vi "DT_Find Next Triangulation_Base Point.vi"(7 "left/right pt (right:F)":bool, 8 "search point":i32, 9 "external point":i32, 10 "Triangles In":i32[][](array[numeric]), 11 "Points In":cluster{"x":dbl, "y":dbl, "index":i32}[](array[cluster])) -> (0 "base point":i32, 1 "triangle":i32, 2 "Triangles Out":i32[][](array[numeric]), 3 "Points Out":cluster{"x":dbl, "y":dbl, "index":i32}[](array[cluster]), 4 "error":i32)   [LabVIEW 2017, in "NI_AAL_Geometry.lvlib"]
uses:
  <vilib>/Analysis/NI_AAL_Geometry.lvlib
  <vilib>/Analysis/geometry.llb/DT_Triangle Manager_Get Adj_by Point.vi
  <vilib>/Analysis/geometry.llb/DT_Triangle Manager_Get Oppo Point_in Ghost.vi
  <vilib>/Analysis/geometry.llb/DT_Triangle Manager_Get Ghost Point.vi
  <vilib>/Analysis/geometry.llb/DT_Triangle Manager_Get Oppo Point.vi
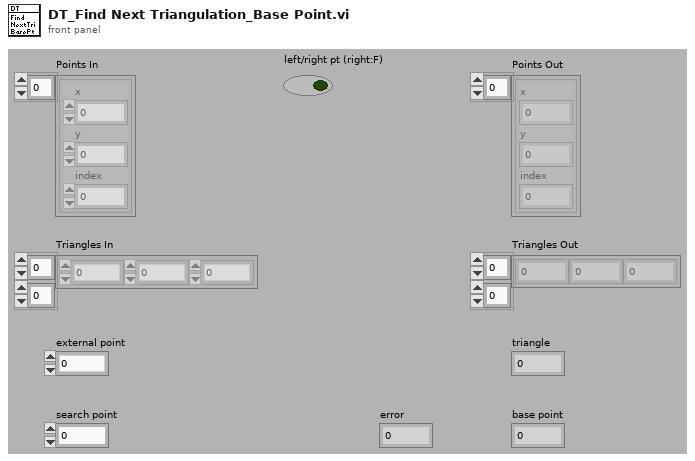
[diagram p1: front panel]
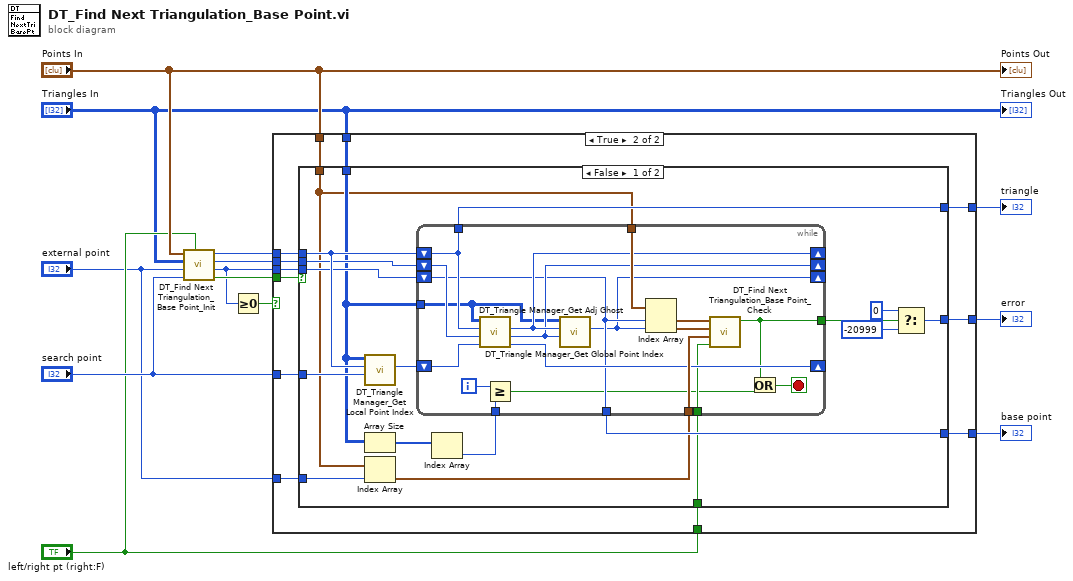
[diagram p0: block diagram]
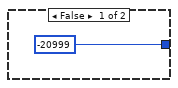
[diagram p2: hidden frame]
diagram:
  n1 = call <vilib>:"DT_Find Next Triangulation_Base Point_Init.vi"("left/right pt (right:F)"="left/right pt (right:F)", "search point"="search point", "external point"="external point", "Triangles In"="Triangles In", "Points In"="Points In") -> ("done?"=w11:bool, "global idx"=w2:i32, "local idx"=w9:i32, "triangle"=w10:i32)  [unwired: 3 in]
  n2 = Greater Or Equal To 0?(x=w2) -> (x >= 0?=w1:bool)
  n3 = case shown="True" w1 {
    tunnel: [_ w26] -> w13
    tunnel: [_ w25] -> w12
    tunnel: w11 -> [_ w24]
    tunnel: w10 -> [_ w23]
    tunnel: w9 -> [_ w22]
    tunnel: w2 -> [_ w21]
    tunnel: "Points In" -> [_ w20]
    tunnel: "search point" -> [_ w19]
    tunnel: "left/right pt (right:F)" -> [_ w18]
    tunnel: "external point" -> [_ w17]
    tunnel: "Triangles In" -> [_ w16]
    tunnel: [-20999 w15] -> w3
    frame False {
    }
    frame True {
      n4 = case shown="False" w24 {
        tunnel: w19 -> [w42 _]
        tunnel: [w44 w64] -> w26
        tunnel: [w41 w65] -> w25
        tunnel: w16 -> [w28 _]
        tunnel: w20 -> [w27 _]
        tunnel: w18 -> [w40 _]
        tunnel: w23 -> [w38 w65]
        tunnel: w22 -> [w37 _]
        tunnel: w21 -> [w36 w64]
        tunnel: w17 -> [w35 _]
        tunnel: [w29 _] -> w15
        frame False {
          n5 = call <vilib>:"DT_Triangle Manager_Get Local Point Index.vi"("global idx"=w42, "triangle"=w38, "Triangles"=w28) -> ("local idx"=w43:i32)  [unwired: 8 out]
          n6 = Array Size(array=w28) -> (size(s)=w34:i32[])
          n7 = Index Array(array=w27, index=w35) -> (element=w39:cluster{"x":dbl, "y":dbl, "index":i32})
          n8 = Index Array(array=w34) -> (element=w33:i32)  [unwired: 1 in]
          n9 = while {
            tunnel: w28 -> [w50]
            tunnel: w27 -> [w63]
            tunnel: w39 -> [w60]
            shift-right: [w51] -> _
            shift-left: w36 -> [w52]
            tunnel: [w52] -> w44
            shift-right: [w59] -> _
            shift-left: w38 -> [w54]
            shift-right: [w55] -> _
            shift-left: w43 -> [w57]
            shift-right: [w56] -> _
            shift-left: w37 -> [w58]
            tunnel: [w54] -> w41
            tunnel: w40 -> [w53]
            tunnel: w33 -> [w47]
            tunnel: [w45] -> w30
            i -> [w49]
            stop <- w48 stop-if-true
            n10 = call <vilib>:"DT_Triangle Manager_Get Adj Ghost.vi"("cur point idx"=w57, "cur base point idx"=w58, "cur triangle"=w54, "Triangles In"=w50) -> ("next point idx"=w55:i32, "next base point idx"=w56:i32, "next triangle"=w59:i32)  [unwired: 5 out]
            n11 = Greater Or Equal?(x=w49, y=w47) -> (x >= y?=w46:bool)
            n12 = call <vilib>:"DT_Triangle Manager_Get Global Point Index.vi"("local idx"=w56, "triangle"=w59, "Triangles"=w50) -> ("global idx"=w51:i32)  [unwired: 8 out]
            n13 = Index Array(array=w63, index #1=w52, index #2=w51) -> (element #1=w62:cluster{"x":dbl, "y":dbl, "index":i32}, element #2=w61:cluster{"x":dbl, "y":dbl, "index":i32})
            n14 = call <vilib>:"DT_Find Next Triangulation_Base Point_Check.vi"("left/right pt (right:F)"=w53, "p 3"=w60, "p 2"=w61, "p 1"=w62) -> ("pass?"=w45:bool)  [unwired: 7 out]
            n15 = Or(x=w45, y=w46) -> (x .or. y?=w48:bool)
          }
          n16 = Select(t=0, s=w30, f=-20999) -> (s? t:f=w29:i32)
        }
        frame True {
        }
      }
    }
  }
  "base point" <- w13
  "triangle" <- w12
  "error" <- w3
  "Points Out" <- "Points In"
  "Triangles Out" <- "Triangles In"
